vi "register.vi"(0 "HGF_SVMonitor":refnum<class "HGF_SVMonitor.lvclass">, 5 "Variable URL":string, 7 "HGF_NetworkVisitor":refnum<class "HGF_NetworkVisitor.lvclass">, 9 "HGF_TriggeredEvent":refnum<class "HGF_TriggeredEvent.lvclass">, 11 "error in (no error)":errorcluster) -> (4 "dup HGF_SVMonitor":refnum<class "HGF_SVMonitor.lvclass">, 15 "error out":errorcluster)   [LabVIEW 2012, in "HGF_SV.lvlib" / "HGF_SVMonitor.lvclass"]
doc: "register a shared variable to the monitor"
uses:
  HGF_SVMonitor.lvclass
  HGF_BaseClasses/HGF_NetworkVisitor/HGF_NetworkVisitor.lvclass
  HGF_BaseClasses/HGF_TriggeredEvent/HGF_TriggeredEvent.lvclass
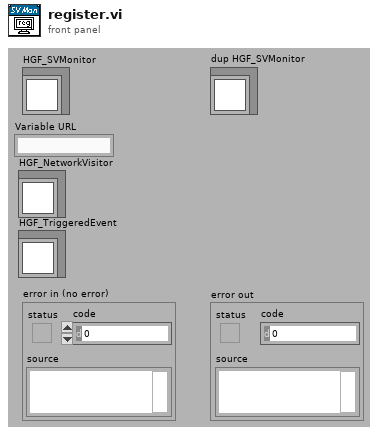
[diagram p1: front panel]
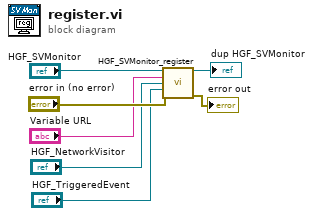
[diagram p0: block diagram]
diagram:
  n1 = call "HGF_SVMonitor_register.vi"("HGF_SVMonitor"="HGF_SVMonitor", "Variable URL"="Variable URL", "HGF_NetworkVisitor"="HGF_NetworkVisitor", "HGF_TriggeredEvent"="HGF_TriggeredEvent", "error in (no error)"="error in (no error)") -> ("HGF_SVMonitor"=→"dup HGF_SVMonitor":refnum<class "HGF_SVMonitor.lvclass">, "error out"=→"error out":errorcluster)  [unwired: 9 in]
